vi "Write Digital Port.vi"(8 "error in (no error)":errorcluster, 10 "DOs":bool[](array[boolean]), 11 "NI Digital Output in":refnum<class "NI DIO.lvclass">) -> (0 "error out":errorcluster, 3 "NI Digital Output out":refnum<class "NI DIO.lvclass">)   [LabVIEW 2025, in "Digital IO.lvlib" / "NI DIO.lvclass"]
uses:
  NI DIO.lvclass
  NI DIO.lvclass/NI DIO.ctl
  <vilib>/DAQmx/write.llb/DAQmx Write (Digital 1D Bool 1Chan 1Samp).vi
  <vilib>/DAQmx/miscellaneous.llb/DAQmx Fill In Error Info.vi
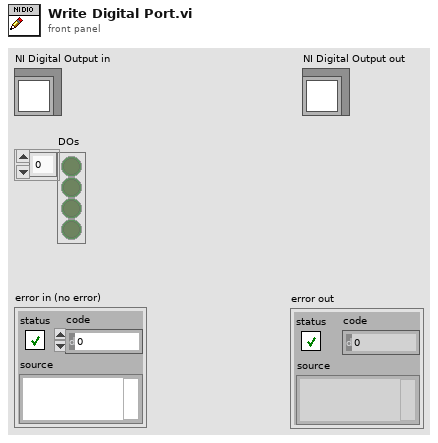
[diagram p1: front panel]
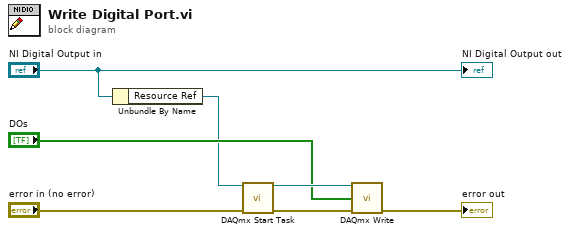
[diagram p0: block diagram]
diagram:
  n1 = Unbundle By Name("NI Digital Output in") -> ("Resource Ref"=w1:refnum<k21>)
  n2 = call <vilib>:"DAQmx Start Task.vi"("task/channels in"=w1, "error in"="error in (no error)") -> ("task out"=w7:refnum<k21>, "error out"=w6:errorcluster)  [unwired: 12 in]
  n3 = call-poly <vilib>:"DAQmx Write.vi"("task/channels in"=w7, "data"="DOs", "error in"=w6) -> ("error out"=→"error out":errorcluster)  [unwired: 10 in, 2 out]
  "NI Digital Output out" <- "NI Digital Output in"
